vi "ProcessWSProtocol.vi"(8 "error in (no error)":errorcluster, 10 "Supported Protocols (any)":string[](array[string]), 11 "Headers In":variant) -> (0 "error out":errorcluster, 3 "Protocol Header":T1[](array[typedef]))   [LabVIEW 2017, in "LV WebSockets.lvlib"]
doc: "Checks the headers for Sec-WebSocket-Protocol and if present, matches against the list of supported protocols specified by the server. If no protocols are supported, this VI will not return an error but the protocol will not returned.\nWebSockets 1.6.0.22\nSam Sharp - MediaMongrels Ltd\nCopyright (c) 2016, MediaMongrels Ltd"
uses:
  LV WebSockets.lvlib
  Headers.ctl
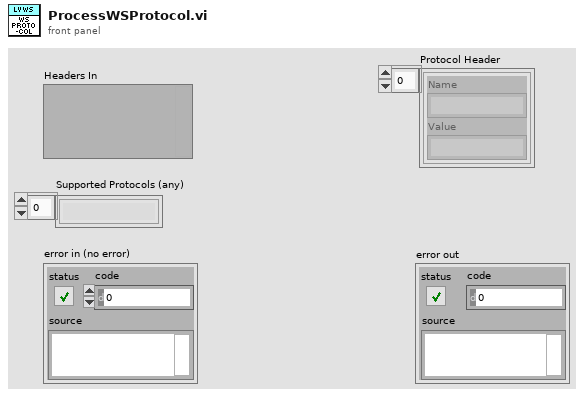
[diagram p1: front panel]
types:
  T1 = typedef "LV WebSockets.lvlib/Headers.ctl" = cluster{"Name":string, "Value":string}
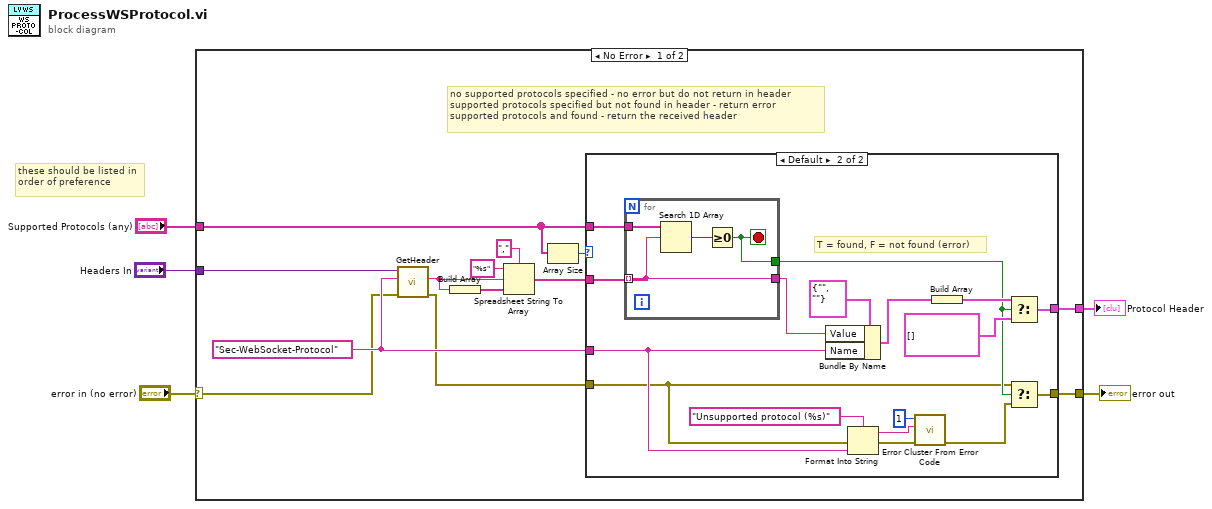
[diagram p0: block diagram]
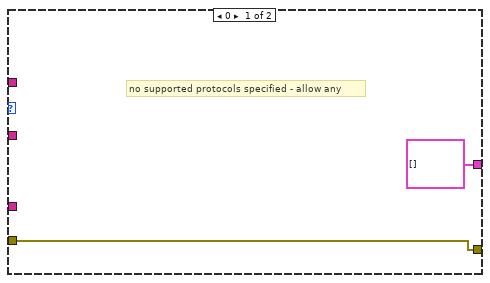
[diagram p2: hidden frame]
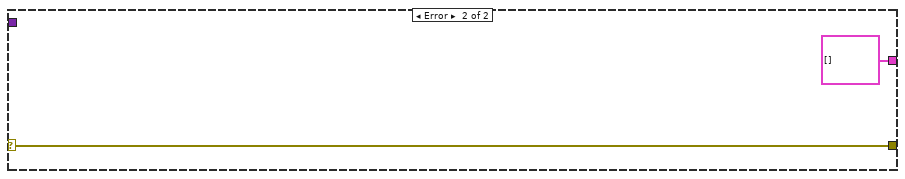
[diagram p3: hidden frame]
diagram:
  # "these should be listed in order of preference"
  n1 = case shown="No Error" "error in (no error)" {
    selector: "error in (no error)" -> [w6 w43]
    tunnel: "Headers In" -> [w18 _]
    tunnel: [w13 T1[] [] ("additional headers (none)")] -> w4
    tunnel: "Supported Protocols (any)" -> [w9 _]
    tunnel: [w7 w43] -> w2
    frame No Error {
      w12 = "Sec-WebSocket-Protocol" ("Name")
      # "no supported protocols specified - no error but do not return in header\nsupported protocols specified but not found in header - return error\nsupported protocols and found - return the received header"
      n2 = call "GetHeader.vi"("error in (no error)"=w6, "Name"=w12, "Headers In"=w18) -> ("error out"=w8:errorcluster, "Data"=w14:string)  [unwired: 5 in, 2 out]
      n3 = Build Array(w14) -> (w15:string[])
      n4 = Spreadsheet String To Array(delimiter (Tab)=",", format string="%s", spreadsheet string=w14, array type (2D Dbl)=w15) -> (array=w11:string[])
      n5 = Array Size(array=w9) -> (size(s)=w10:i32)
      n6 = case shown="Default" w10 {
        tunnel: w9 -> [_ w37]
        tunnel: w11 -> [_ w36]
        tunnel: [T1[] [] ("additional headers (none)") w34] -> w13
        tunnel: w12 -> [_ w26]
        tunnel: w8 -> [w19 w25]
        tunnel: [w19 w28] -> w7
        frame 0 {
          # "no supported protocols specified - allow any"
        }
        frame Default {
          # "T = found, F = not found (error)"
          n7 = for {
            tunnel: w36 -> [w40] mode=indexing
            tunnel: w37 -> [w41]
            tunnel: [w40] -> w32
            tunnel: [w38] -> w29
            stop <- w38 stop-if-true
            n8 = Search 1D Array(1D array=w41, element=w40) -> (index of element=w39:i32)  [unwired: 1 in]
            n9 = Greater Or Equal To 0?(x=w39) -> (x >= 0?=w38:bool)
          }
          n10 = Bundle By Name(cluster=T1 {"Name"="", "Value"=""}, "Value"=w32, "Name"=w26) -> (w31:T1)
          n11 = Format Into String(format string="Unsupported protocol (%s)", error in=w25, w26) -> (resulting string=w22:string, error out=w24:errorcluster)  [unwired: 1 in]
          n12 = call <vilib>:"Error Cluster From Error Code.vi"("error in (no error)"=w24, "error message (\"\")"=w22, "error code (0)"=1) -> ("error out"=w23:errorcluster)  [unwired: 6 in]
          n13 = Build Array(w31) -> (w30:T1[])
          n14 = Select(t=w30, s=w29, f=T1[] [] ("additional headers (none)")) -> (s? t:f=w34:T1[])
          n15 = Select(t=w25, s=w29, f=w23) -> (s? t:f=w28:errorcluster)
        }
      }
    }
    frame Error {
    }
  }
  "Protocol Header" <- w4
  "error out" <- w2
